vi "Update Console.vi"(0 "New Line":string, 2 "Function":T1, 7 "Console Ref":refnum<vi>, 11 "Error In":errorcluster) -> (4 "Existing String":string, 15 "Error Out":errorcluster)   [LabVIEW 2021]
doc: "Appends the input string as a new line to the reference console string."
uses:
  Controls/Console Manager Functions.ctl
panel:
  # "Inputs"
  # "Outputs"
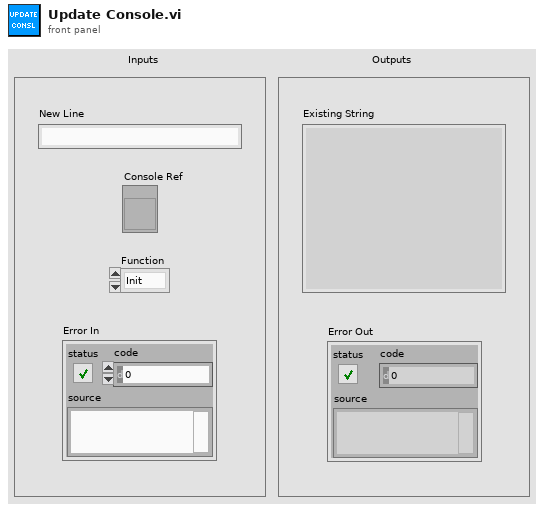
[diagram p1: front panel]
types:
  T1 = typedef "Console Manager Functions.ctl" = enum16{"Init", "Add", "Get"}
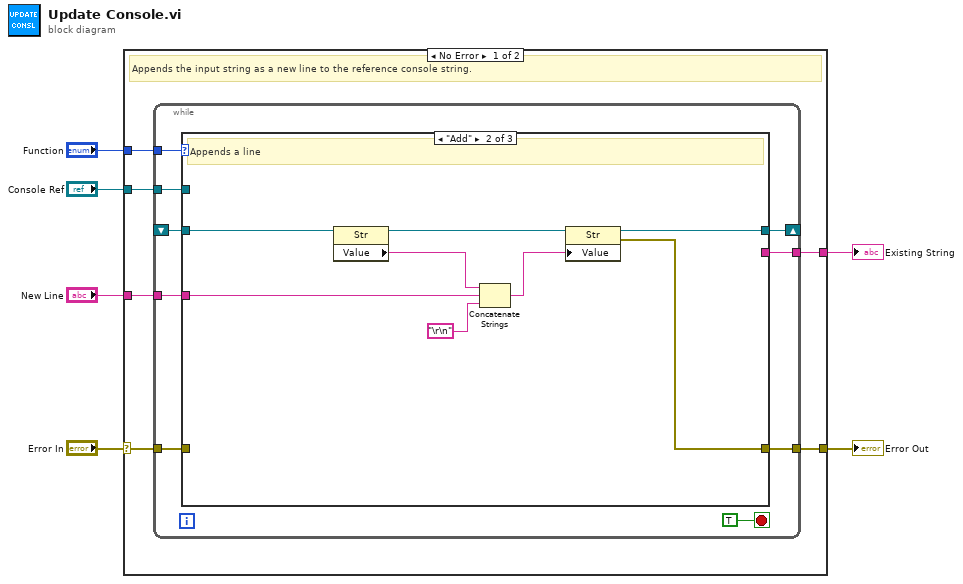
[diagram p0: block diagram]
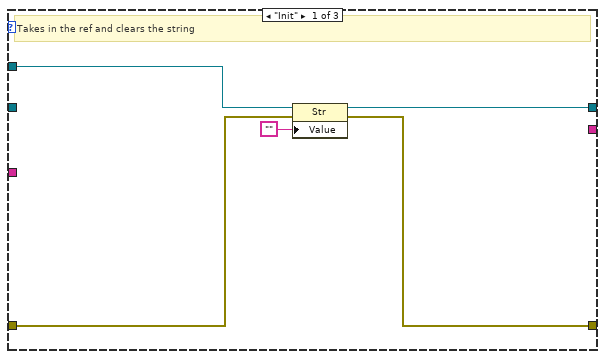
[diagram p2: hidden frame]
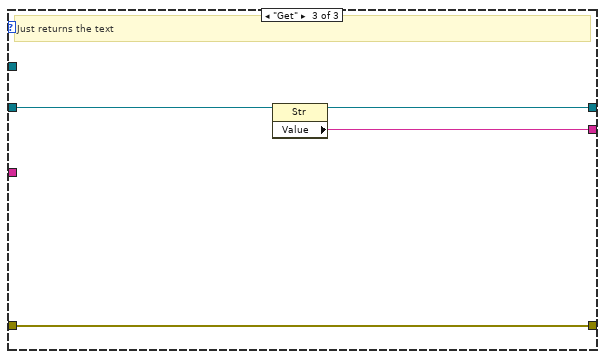
[diagram p3: hidden frame]
diagram:
  n1 = case shown="No Error" "Error In" {
    selector: "Error In" -> [w8 w39]
    tunnel: "New Line" -> [w12 _]
    tunnel: "Console Ref" -> [w11 _]
    tunnel: "Function" -> [w10 _]
    tunnel: [w9 w39] -> w2
    tunnel: [w7 _] -> w1
    frame No Error {
      # "Appends the input string as a new line to the reference console string."
      n2 = while {
        tunnel: w12 -> [w21]
        tunnel: w11 -> [w20]
        tunnel: w10 -> [w19]
        shift-right: [w18] -> _
        shift-left: _ -> [w14]
        tunnel: [w16] -> w9
        tunnel: w8 -> [w15]
        tunnel: [w13] -> w7
        stop <- TRUE stop-if-true
        n3 = case shown="\"Add\"" w19 {
          tunnel: w21 -> [_ w27 _]
          tunnel: w20 -> [w26 _ _]
          tunnel: [w25 w32 w36] -> w18
          tunnel: [w23 w31 w38] -> w16
          tunnel: w15 -> [w22 _ w38]
          tunnel: w14 -> [_ w34 w37]
          tunnel: [_ _ w35] -> w13
          frame "Init" {
            # "Takes in the ref and clears the string"
            n4 = property class="Str"(reference=w26, error in=w22, "Value"="") -> (reference out=w25:refnum<vi>, error out=w23:errorcluster)
          }
          frame "Add" {
            # "Appends a line"
            n5 = property class="Str"(reference=w34) -> (reference out=w33:refnum<vi>, "Value"=w30:string)  [unwired: 1 in, 1 out]
            n6 = Concatenate Strings(w30, w27, "\r\n") -> (w29:string)
            n7 = property class="Str"(reference=w33, "Value"=w29) -> (reference out=w32:refnum<vi>, error out=w31:errorcluster)  [unwired: 1 in]
          }
          frame "Get" {
            # "Just returns the text"
            n8 = property class="Str"(reference=w37) -> (reference out=w36:refnum<vi>, "Value"=w35:string)  [unwired: 1 in, 1 out]
          }
        }
      }
    }
    frame Error {
      # "Can't start due to error"
    }
  }
  "Error Out" <- w2
  "Existing String" <- w1
